vi "ADCP_read_data_packet_from_serial_port.vi"(8 "error in (no error)":errorcluster, 9 "Timeout interval (ms)":u32, 10 "Frame Name":string, 11 "ADCP In":refnum<class "ADCP.lvclass">) -> (0 "error out":errorcluster, 3 "ADCP out":refnum<class "ADCP.lvclass">)   [LabVIEW 2017, in "ADCP.lvclass"]
uses:
  ADCP.lvclass
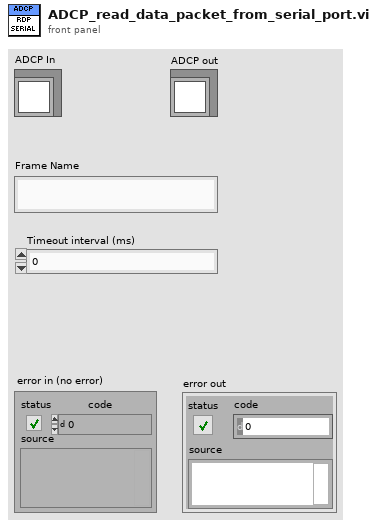
[diagram p1: front panel]
types:
  T1 = enum16{"Data", "Connection Management", "Remote Request", "Error and status", "INVALID"}
  T2 = typedef "ADCP.lvclass/ADCP_Data_Packet_Transmit_Mode.ctl" = enum16{"Disable", "Single", "Cyclic", "Repeat"}
  T3 = cluster{"Parameters":cluster{"Parameter name":string, "Node name":string, "Node ID":u8, "Frame name":string, "Frame ID":u8, "Start bit":u32, "Bit length":u32, "Factor":dbl, "Offset":dbl, "Minimum":dbl, "Maximum":dbl, "Value":string, "Comments":string, "Data_Type":enum16{"BOOL", "UNSIGNED", "SIGNED", "FLOAT32", "ENUM"}, "Enum List":string[]}[], "Priority":enum16{"LOW", "HIGH"}, "Node name":string, "Node ID":u8, "Frame name":string, "Frame ID":u8, "Data":u32, "Raw bytes":u8[], "Processed bytes":u8[], "Tx count":i32, "Last Tx Time":u32, "Tx interval":u32, "Rx count":i32, "Last Rx Time":u32, "Rx interval":u32, "Tx Enable":bool, "Tx mode":T2, "Repeat/Cyclic Tx interval":u32, "Repeat count":u16}
  T4 = typedef "ADCP.lvclass/ADCP_Packet_Info.ctl" = cluster{"Priority":enum16{"LOW", "HIGH"}, "Type":enum16{"Data", "Connection Management", "Remote Request", "Error and status", "INVALID"}, "Node ID":i32, "Frame ID":i32, "Checksum valid ?":bool, "Current time (ms)":u32}
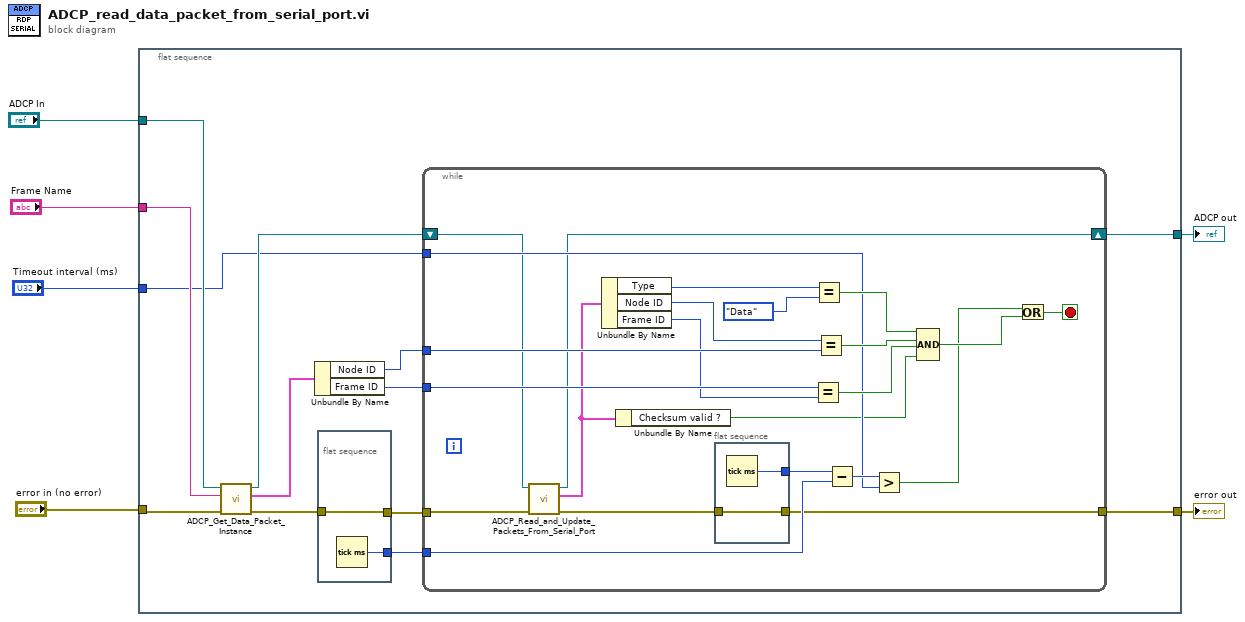
[diagram p0: block diagram]
diagram:
  n1 = flat-sequence {
    tunnel: "ADCP In" -> [w18]
    tunnel: "Frame Name" -> [w17]
    tunnel: "Timeout interval (ms)" -> [w9]
    tunnel: "error in (no error)" -> [w19]
    tunnel: [w8] -> w1
    tunnel: [w7] -> w2
    frame #0 {
      n2 = call "ADCP_Get_Data_Packet_Instance.vi"("error in (no error)"=w19, "Frame name"=w17, "ADCP in"=w18) -> ("error out"=w15:errorcluster, "Data Packet"=w16:T3, "ADCP out"=w13:refnum<class "ADCP.lvclass">)  [unwired: 6 in]
      n3 = Unbundle By Name(w16) -> ("Node ID"=w12:u8, "Frame ID"=w11:u8)
      n4 = flat-sequence {
        tunnel: w15 -> [w46]
        tunnel: [w46] -> w14
        tunnel: [w45] -> w10
        frame #0 {
          n5 = Tick Count (ms)() -> (millisecond timer value=w45:u32)
        }
      }
      n6 = while {
        tunnel: w14 -> [w29]
        tunnel: w12 -> [w41]
        tunnel: w11 -> [w40]
        tunnel: w10 -> [w34]
        tunnel: w9 -> [w32]
        tunnel: [w23] -> w8
        shift-right: [w22] -> w7
        shift-left: w13 -> [w28]
        stop <- w30 stop-if-true
        n7 = call "ADCP_Read_and_Update_Packets_From_Serial_Port.vi"("error in (no error)"=w29, "ADCP In"=w28) -> ("error out"=w24:errorcluster, "Packet Info"=w21:T4, "ADCP out"=w22:refnum<class "ADCP.lvclass">)  [unwired: 6 in, 1 out]
        n8 = Unbundle By Name(w21) -> ("Type"=w27:T1, "Node ID"=w26:i32, "Frame ID"=w25:i32)
        n9 = Unbundle By Name(w21) -> ("Checksum valid ?"=w20:bool)
        n10 = flat-sequence {
          tunnel: [w44] -> w35
          tunnel: w24 -> [w43]
          tunnel: [w43] -> w23
          frame #0 {
            n11 = Tick Count (ms)() -> (millisecond timer value=w44:u32)
          }
        }
        n12 = Equal?(x=w40, y=w25) -> (x = y?=w37:bool)
        n13 = Equal?(x=w27, y=T1."Data") -> (x = y?=w39:bool)
        n14 = Equal?(x=w26, y=w41) -> (x = y?=w38:bool)
        n15 = Subtract(x=w35, y=w34) -> (x-y=w33:u32)
        n16 = Greater?(x=w33, y=w32) -> (0:w31:bool)
        n17 = Compound Arithmetic op=AND(w39, w38, w37, w20) -> (w36:bool)
        n18 = Or(x=w31, y=w36) -> (x .or. y?=w30:bool)
      }
    }
  }
  "ADCP out" <- w2
  "error out" <- w1
